vi "Remote_Request_Frame_Test.vi"() -> ()   [LabVIEW 2017]
uses:
  Classes/ADCP_Data_Packet_Transmit_Mode.ctl
  Classes/ADCP.lvclass
panel:
  out "Data Packets":T2(array[cluster])
  in  "Request Frame IDs":u8[](array[numeric])
  in  "Symbol File Path":path
  in  "ADCP Session Parameters":T3
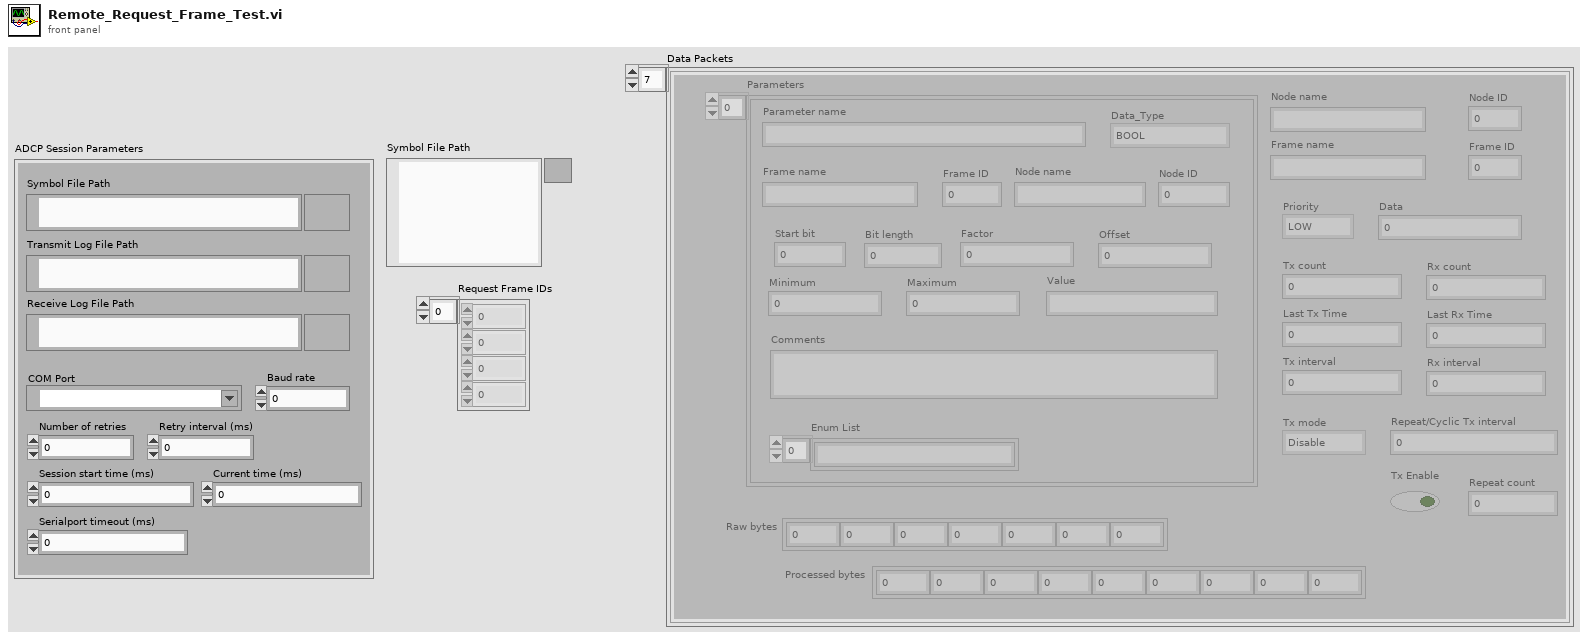
[diagram p1: front panel]
types:
  T1 = typedef "ADCP.lvclass/ADCP_Data_Packet_Transmit_Mode.ctl" = enum16{"Disable", "Single", "Cyclic", "Repeat"}
  T2 = cluster{"Parameters":cluster{"Parameter name":string, "Node name":string, "Node ID":u8, "Frame name":string, "Frame ID":u8, "Start bit":u32, "Bit length":u32, "Factor":dbl, "Offset":dbl, "Minimum":dbl, "Maximum":dbl, "Value":string, "Comments":string, "Data_Type":enum16{"BOOL", "UNSIGNED", "SIGNED", "FLOAT32", "ENUM"}, "Enum List":string[]}[], "Priority":enum16{"LOW", "HIGH"}, "Node name":string, "Node ID":u8, "Frame name":string, "Frame ID":u8, "Data":u32, "Raw bytes":u8[], "Processed bytes":u8[], "Tx count":i32, "Last Tx Time":u32, "Tx interval":u32, "Rx count":i32, "Last Rx Time":u32, "Rx interval":u32, "Tx Enable":bool, "Tx mode":T1, "Repeat/Cyclic Tx interval":u32, "Repeat count":u16}[]
  T3 = cluster{"Symbol File Path":path, "Transmit Log File Path":path, "Receive Log File Path":path, "COM Port":refnum<visa-resource-name>, "Baud rate":u32, "Number of retries":u16, "Retry interval (ms)":u16, "Session start time (ms)":u32, "Current time (ms)":u32, "Serialport timeout (ms)":u32}
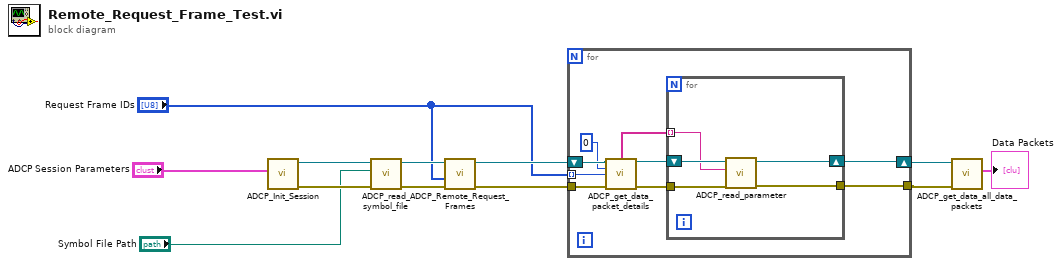
[diagram p0: block diagram]
diagram:
  n1 = call "ADCP_Init_Session.vi"("ADCP Session Parameters"="ADCP Session Parameters") -> ("error out"=w10:errorcluster, "ADCP out"=w11:refnum<class "ADCP.lvclass">)  [unwired: 9 in]
  n2 = call "ADCP_read_symbol_file.vi"("error in (no error)"=w10, "Symbol File Path"="Symbol File Path", "ADCP in"=w11) -> ("error out"=w7:errorcluster, "ADCP out"=w8:refnum<class "ADCP.lvclass">)  [unwired: 5 in, 2 out]
  n3 = call "ADCP_Remote_Request_Frames.vi"("error in (no error)"=w7, "Request Frame IDs"="Request Frame IDs", "ADCP In"=w8) -> ("error out"=w5:errorcluster, "ADCP Out"=w6:refnum<class "ADCP.lvclass">)  [unwired: 7 in]
  n4 = for {
    tunnel: w5 -> [w20]
    tunnel: "Request Frame IDs" -> [w18] mode=indexing
    shift-right: [w15] -> w2
    shift-left: w6 -> [w21]
    tunnel: [w13] -> w3
    n5 = call "ADCP_get_data_packet_details.vi"("ADCP In"=w21, "NID"=u8 0, "FID"=w18, "error in (no error)"=w20) -> ("Parameter names"=w14:string[], "ADCP Out"=w16:refnum<class "ADCP.lvclass">, "error out"=w17:errorcluster)  [unwired: 5 in, 4 out]
    n6 = for {
      tunnel: w17 -> [w25]
      shift-right: [w24] -> w15
      shift-left: w16 -> [w26]
      tunnel: w14 -> [w23] mode=indexing
      tunnel: [w22] -> w13
      n7 = call "ADCP_read_parameter.vi"("error in (no error)"=w25, "Parameter Name"=w23, "ADCP In"=w26) -> ("error out"=w22:errorcluster, "ADCP out"=w24:refnum<class "ADCP.lvclass">)  [unwired: 5 in, 2 out]
    }
  }
  n8 = call "ADCP_get_data_all_data_packets.vi"("error in (no error)"=w3, "ADCP In"=w2) -> ("Data Packets"=→"Data Packets":T2)  [unwired: 7 in, 2 out]
